vi "Update Outgoing Section.vi"(8 "error in (no error)":errorcluster, 10 "Outgoing":T2 {"Frames to Update"."Node Ref" format="%.0x"; "Frames to Delete" format="%.0x"}, 11 "Item Ref in":T1 format="%.0x") -> (0 "error out":errorcluster, 3 "Item Ref out":T1 format="%.0x")   [LabVIEW 2025, in "Protection and Counter Addon System Explorer.lvlib"]
uses:
  Protection and Counter Addon System Explorer.lvlib
  Types/VS Update List.ctl
  <vilib>/NI VeriStand/Custom Device API/Custom Device Item Ref.ctl
  Types/Base Frame Info_NoVS.ctl
  Types/Signal Attributes.ctl
  Types/CAN Filter Type.ctl
  Types/CAN Frame Update Results.ctl
  <vilib>/NI VeriStand/Custom Device Tools/Custom Device Utility Library/Search Direction.ctl
  <vilib>/NI VeriStand/Custom Device API/Custom Device Channel.ctl
  <vilib>/NI VeriStand/Custom Device API/Custom Device Channel Type.ctl
  Addon Shared/SubVIs/GUID Lookup.vi
  <vilib>/NI/NI VeriStand Advanced SysDef API/_SubVIs/SysDef.Property.Set.U32.vi
  <vilib>/NI/NI VeriStand Advanced SysDef API/_SubVIs/SysDef.Search.Name.vi
  <vilib>/NI VeriStand/Custom Device Tools/Custom Device Utility Library/NI VeriStand - Search for Item by GUID.vi
  <vilib>/NI/NI VeriStand Advanced SysDef API/SysDef API/Advanced System Definition.lvlib
  Addon Shared/Protection and Counter Addon Shared.lvlib
  <vilib>/NI VeriStand/Custom Device API/Custom Device API.lvlib
  <vilib>/NI VeriStand/Custom Device Tools/Custom Device Utility Library/Custom Device Utility Library.lvlib
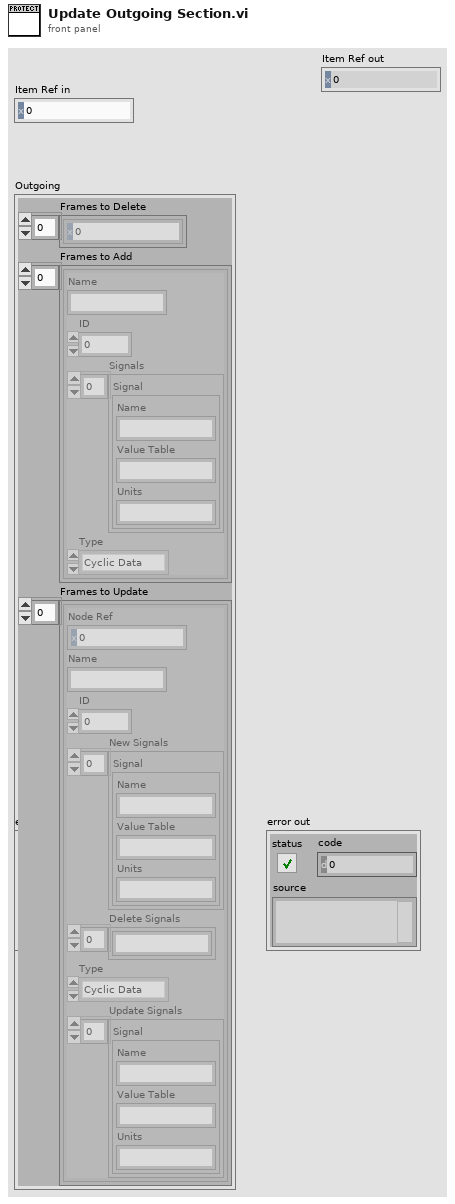
[diagram p1: front panel]
types:
  T1 = typedef "Custom Device API.lvlib/Custom Device Item Ref.ctl" = u64
  T2 = typedef "Protection and Counter Addon System Explorer.lvlib/VS Update List.ctl" = cluster{"Frames to Delete":T1[], "Frames to Add":T3[], "Frames to Update":T6[]}
  T3 = typedef "Protection and Counter Addon System Explorer.lvlib/Base Frame Info_NoVS.ctl" = cluster{"Name":string, "ID":u32, "Signals":T4[], "Type":T5}
  T4 = typedef "Protection and Counter Addon System Explorer.lvlib/Signal Attributes.ctl" = cluster{"Name":string, "Value Table":string, "Units":string}
  T5 = typedef "Protection and Counter Addon System Explorer.lvlib/CAN Filter Type.ctl" = enum16{"Cyclic Data", "Event Data", "Cyclic/Event", "All"}
  T6 = typedef "Protection and Counter Addon System Explorer.lvlib/CAN Frame Update Results.ctl" = cluster{"Node Ref":T1, "Name":string, "ID":u32, "New Signals":T4[], "Delete Signals":string[], "Type":T5, "Update Signals":T4[]}
  T7 = typedef "Custom Device Utility Library.lvlib/Search Direction.ctl" = enum16{"Down", "Up"}
  T8 = typedef "Custom Device API.lvlib/Custom Device Channel.ctl" = cluster{"Type":T9, "Units":string, "Default Value":dbl, "Faultable":bool, "Scalable":bool}
  T9 = typedef "Custom Device API.lvlib/Custom Device Channel Type.ctl" = enum16{"Input", "Output"}
  T10 = typedef "Custom Device API.lvlib/Custom Device Item Info.ctl" = cluster{"Name":string, "Is Channel":bool, "GUID":string, "Is Waveform":bool}
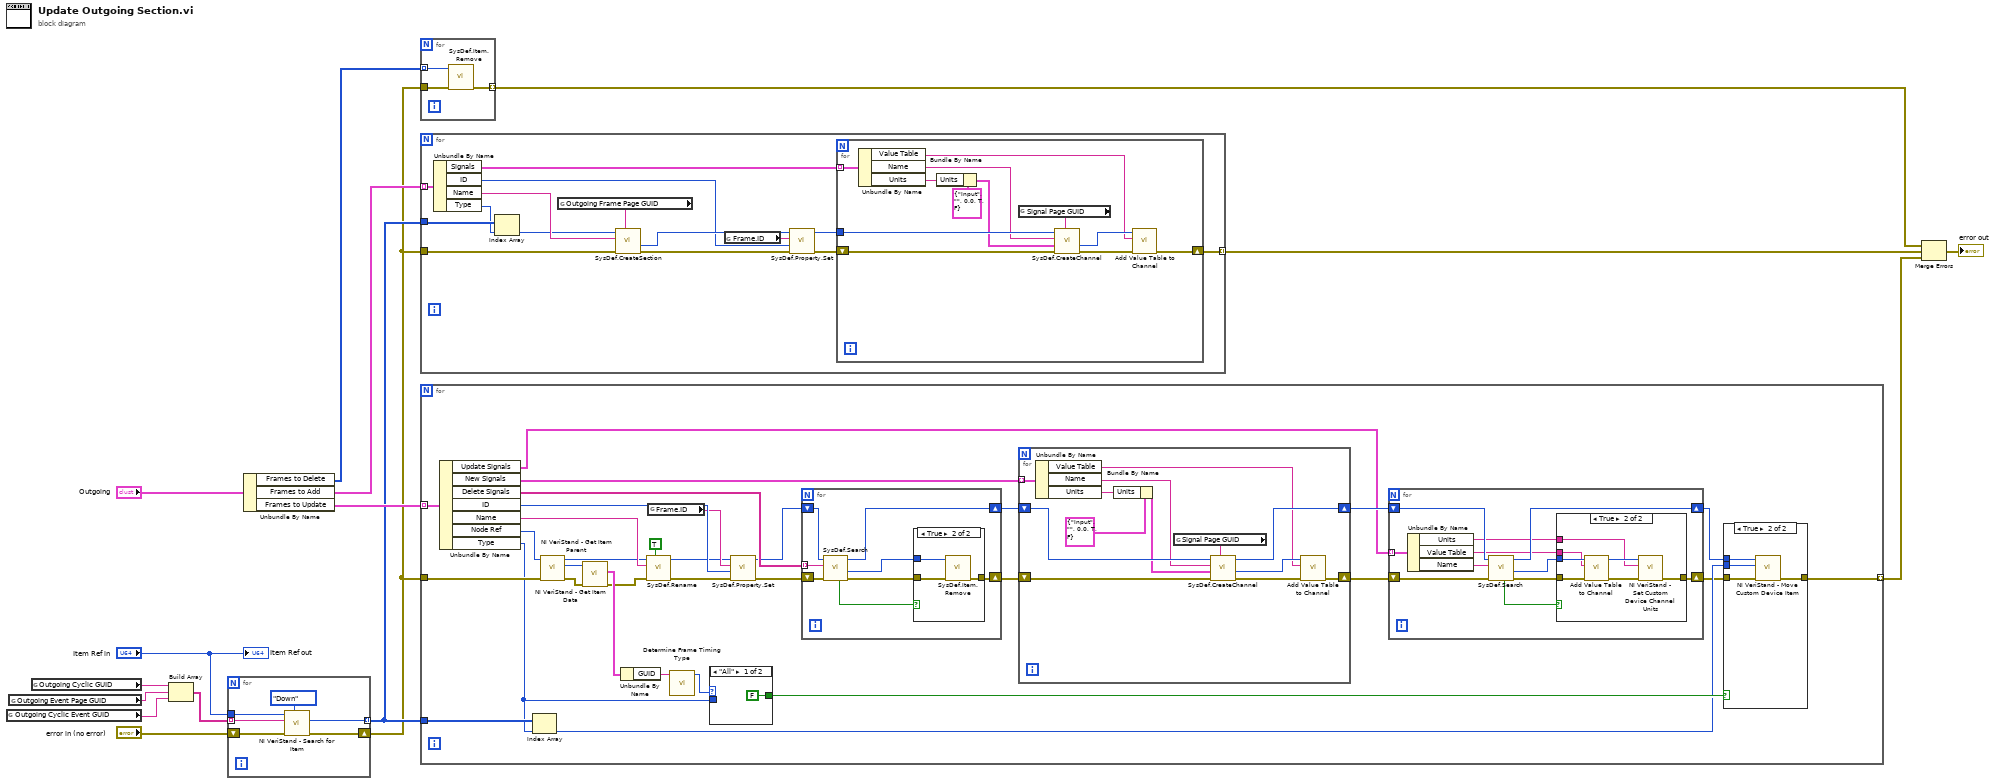
[diagram p0: block diagram]
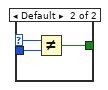
[diagram p2: hidden frame]
diagram:
  n1 = global read "GUID Lookup.vi" "Outgoing Cyclic Event GUID"() -> (w6:string)
  n2 = global read "GUID Lookup.vi" "Outgoing Event Page GUID"() -> (w5:string)
  n3 = global read "GUID Lookup.vi" "Outgoing Cyclic GUID"() -> (w4:string)
  n4 = Build Array(w4, w5, w6) -> (w8:string[])
  n5 = for {
    tunnel: "Item Ref in" -> [w21]
    tunnel: w8 -> [w20] mode=indexing
    shift-right: [w18] -> w3
    shift-left: "error in (no error)" -> [w19]
    tunnel: [w17] -> w9 mode=indexing
    n6 = call-poly <vilib>:"NI VeriStand - Search for Item.vi"("Direction (Down)"=Search_Direction."Down", "error in"=w19, "Item GUID"=w20, "Section Ref in"=w21) -> ("error out"=w18:errorcluster, "Item Ref"=w17:T1)  [unwired: 4 in, 2 out]
  }
  n7 = Unbundle By Name("Outgoing") -> ("Frames to Delete"=w2:T1[], "Frames to Add"=w15:T3[], "Frames to Update"=w14:T6[])
  n8 = for {
    tunnel: w2 -> [w23] mode=indexing
    tunnel: w3 -> [w25]
    tunnel: [w24] -> w1 mode=indexing
    n9 = call <vilib>:"SysDef.Item.Remove.vi"("error in (no error)"=w25, "nodeID"=w23) -> ("error out"=w24:errorcluster)  [unwired: 8 in, 1 out]
  }
  n10 = for {
    tunnel: w15 -> [w40] mode=indexing
    tunnel: w9 -> [w39]
    tunnel: w3 -> [w27]
    tunnel: [w26] -> w10 mode=indexing
    n11 = Unbundle By Name(w40) -> ("Signals"=w31:T4[], "ID"=w36:u32, "Name"=w34:string, "Type"=w38:T5)
    n12 = Index Array(array=w39, index=w38) -> (element=w28:T1)
    n13 = global read "GUID Lookup.vi" "Outgoing Frame Page GUID"() -> (w29:string)
    n14 = call <vilib>:"SysDef.CreateSection.vi"("GUID"=w29, "error in (no error)"=w27, "Name"=w34, "nodeID"=w28) -> ("error out"=w35:errorcluster, "New NodeID"=w37:u64)  [unwired: 4 in, 2 out]
    n15 = global read "GUID Lookup.vi" "Frame.ID"() -> (w30:string)
    n16 = call-poly <vilib>:"SysDef.Property.Set.vi"("error in (no error)"=w35, "Value"=w36, "Property Name"=w30, "nodeID"=w37) -> ("error out"=w32:errorcluster, "nodeID out"=w33:u64)  [unwired: 6 in]
    n17 = for {
      tunnel: w33 -> [w52]
      tunnel: w31 -> [w50] mode=indexing
      shift-right: [w46] -> w26
      shift-left: w32 -> [w51]
      n18 = Unbundle By Name(w50) -> ("Value Table"=w44:string, "Name"=w48:string, "Units"=w43:string)
      n19 = Bundle By Name(cluster=T8 {"Type"=enum."Input", "Units"="", "Default Value"=0.0, "Faultable"=TRUE, "Scalable"=FALSE} ("Channel"), "Units"=w43) -> (w41:T8)
      n20 = global read "GUID Lookup.vi" "Signal Page GUID"() -> (w49:string)
      n21 = call <vilib>:"SysDef.CreateChannel.vi"("GUID"=w49, "error in (no error)"=w51, "Channel"=w41, "Name"=w48, "nodeID"=w52) -> ("error out"=w47:errorcluster, "New NodeID"=w45:u64)  [unwired: 3 in, 2 out]
      n22 = call "Add Value Table to Channel.vi"("error in (no error)"=w47, "Value Table"=w44, "Channel Ref"=w45) -> ("error out"=w46:errorcluster)  [unwired: 7 in, 1 out]
    }
  }
  n23 = for {
    tunnel: w14 -> [w84] mode=indexing
    tunnel: w9 -> [w71]
    tunnel: w3 -> [w73]
    tunnel: [w62] -> w11 mode=indexing
    n24 = Unbundle By Name(w84) -> ("Update Signals"=w53:T4[], "New Signals"=w79:T4[], "Delete Signals"=w80:string[], "ID"=w82:u32, "Name"=w83:string, "Node Ref"=w74:T1, "Type"=w70:T5)
    n25 = Index Array(array=w71, index=w70) -> (element=w60:T1)
    n26 = call <vilib>:"NI VeriStand - Get Item Parent.vi"("error in (no error)"=w73, "Item Ref in"=w74) -> ("error out"=w77:errorcluster, "Parent Ref"=w78:T1, "Item Ref out"=w58:T1)  [unwired: 6 in, 1 out]
    n27 = call <vilib>:"NI VeriStand - Get Item Data.vi"("error in (no error)"=w77, "Item Ref in"=w78) -> ("error out"=w59:errorcluster, "Item Info"=w76:T10)  [unwired: 6 in, 2 out]
    n28 = Unbundle By Name(w76) -> ("GUID"=w75:string)
    n29 = call <vilib>:"SysDef.Rename.vi"("Force Rename (F)"=TRUE, "error in (no error)"=w59, "Name"=w83, "nodeID"=w58) -> ("error out"=w68:errorcluster, "nodeID out"=w69:u64)  [unwired: 5 in, 1 out]
    n30 = global read "GUID Lookup.vi" "Frame.ID"() -> (w81:string)
    n31 = call "Determine Frame Timing Type.vi"("GUID"=w75) -> ("CAN:Frame Type"=w72:T5)  [unwired: 10 in]
    n32 = case shown="\"All\"" w72 {
      selector: w72 -> [_ w86]
      tunnel: w70 -> [_ w88]
      tunnel: [FALSE w87] -> w61
      frame "All" {
      }
      frame Default {
        n33 = Not Equal?(x=w86, y=w88) -> (x != y?=w87:bool)
      }
    }
    n34 = call-poly <vilib>:"SysDef.Property.Set.vi"("error in (no error)"=w68, "Value"=w82, "Property Name"=w81, "nodeID"=w69) -> ("error out"=w64:errorcluster, "nodeID out"=w67:u64)  [unwired: 6 in]
    n35 = for {
      tunnel: w80 -> [w102] mode=indexing
      shift-right: [w105] -> w66
      shift-left: w67 -> [w109]
      shift-right: [w104] -> w65
      shift-left: w64 -> [w103]
      n36 = call-poly <vilib>:"SysDef.Search.vi"("error in (no error)"=w103, "Name"=w102, "nodeID"=w109) -> ("error out"=w106:errorcluster, "Value out"=w107:u64, "nodeID out"=w105:u64, "Found?"=w108:bool)  [unwired: 5 in]
      n37 = case shown="True" w108 {
        tunnel: w107 -> [_ w113]
        tunnel: w106 -> [w110 w112]
        tunnel: [w110 w111] -> w104
        frame False {
        }
        frame True {
          n38 = call <vilib>:"SysDef.Item.Remove.vi"("error in (no error)"=w112, "nodeID"=w113) -> ("error out"=w111:errorcluster)  [unwired: 8 in, 1 out]
        }
      }
    }
    n39 = for {
      shift-right: [w94] -> w57
      shift-left: w65 -> [w100]
      tunnel: w79 -> [w97] mode=indexing
      shift-right: [w98] -> w55
      shift-left: w66 -> [w101]
      n40 = Unbundle By Name(w97) -> ("Value Table"=w92:string, "Name"=w96:string, "Units"=w91:string)
      n41 = Bundle By Name(cluster=T8 {"Type"=enum."Input", "Units"="", "Default Value"=0.0, "Faultable"=TRUE, "Scalable"=FALSE} ("Channel"), "Units"=w91) -> (w89:T8)
      n42 = global read "GUID Lookup.vi" "Signal Page GUID"() -> (w99:string)
      n43 = call <vilib>:"SysDef.CreateChannel.vi"("GUID"=w99, "error in (no error)"=w100, "Channel"=w89, "Name"=w96, "nodeID"=w101) -> ("error out"=w95:errorcluster, "New NodeID"=w93:u64, "nodeID out"=w98:u64)  [unwired: 3 in, 1 out]
      n44 = call "Add Value Table to Channel.vi"("error in (no error)"=w95, "Value Table"=w92, "Channel Ref"=w93) -> ("error out"=w94:errorcluster)  [unwired: 7 in, 1 out]
    }
    n45 = for {
      tunnel: w53 -> [w117] mode=indexing
      shift-right: [w120] -> w54
      shift-left: w55 -> [w124]
      shift-right: [w119] -> w56
      shift-left: w57 -> [w118]
      n46 = Unbundle By Name(w117) -> ("Units"=w114:string, "Value Table"=w115:string, "Name"=w116:string)
      n47 = call-poly <vilib>:"SysDef.Search.vi"("error in (no error)"=w118, "Name"=w116, "nodeID"=w124) -> ("error out"=w121:errorcluster, "Value out"=w122:u64, "nodeID out"=w120:u64, "Found?"=w123:bool)  [unwired: 5 in]
      n48 = case shown="True" w123 {
        tunnel: w122 -> [_ w131]
        tunnel: w121 -> [w125 w132]
        tunnel: [w125 w127] -> w119
        tunnel: w115 -> [_ w130]
        tunnel: w114 -> [_ w126]
        frame False {
        }
        frame True {
          n49 = call "Add Value Table to Channel.vi"("error in (no error)"=w132, "Value Table"=w130, "Channel Ref"=w131) -> ("error out"=w128:errorcluster, "Channel Ref out"=w129:u64)  [unwired: 7 in]
          n50 = call <vilib>:"NI VeriStand - Set Custom Device Channel Units.vi"("error in (no error)"=w128, "Units"=w126, "Channel Ref in"=w129) -> ("error out"=w127:errorcluster)  [unwired: 7 in, 1 out]
        }
      }
    }
    n51 = case shown="True" w61 {
      tunnel: w56 -> [w133 w137]
      tunnel: w54 -> [_ w135]
      tunnel: [w133 w136] -> w62
      tunnel: w60 -> [_ w134]
      frame False {
      }
      frame True {
        n52 = call <vilib>:"NI VeriStand - Move Custom Device Item.vi"("error in (no error)"=w137, "New Parent Ref in"=w134, "Item Ref in"=w135) -> ("error out"=w136:errorcluster)  [unwired: 6 in, 2 out]
      }
    }
  }
  n53 = Merge Errors(w1, w10, w11) -> (→"error out":errorcluster)
  "Item Ref out" <- "Item Ref in"
